vi "Read Step State.vi"(8 "error in (no error)":errorcluster, 11 "Base Step in":refnum<class "Base Step.lvclass">) -> (0 "error out":errorcluster, 2 "Step State":T1={"Result"="N/A", "Status"="IDLE", "Enabled"=TRUE, "Upper"="", "Target"="", "Lower"="", "Value"=""}, 3 "Base Step out":refnum<class "Base Step.lvclass">)   [LabVIEW 2024, in "Ramses Sequencer.lvlib" / "Base Step.lvclass"]
uses:
  Base Step.lvclass
  Typedefs/Step State.ctl
  Base Step.lvclass/Base Step.ctl
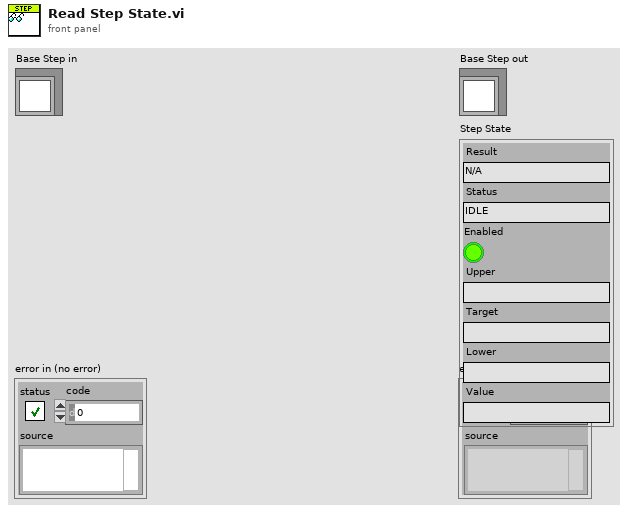
[diagram p1: front panel]
types:
  T1 = typedef "Ramses Sequencer.lvlib/Base Step.lvclass/Step State.ctl" = cluster{"Result":string, "Status":string, "Enabled":bool, "Upper":string, "Target":string, "Lower":string, "Value":string}
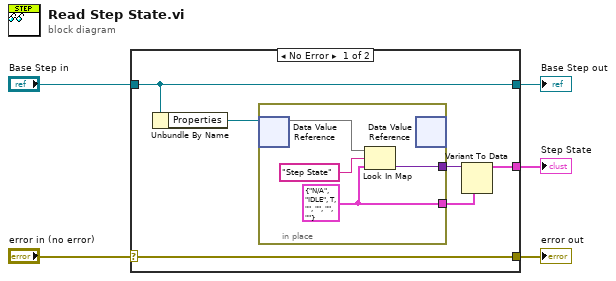
[diagram p0: block diagram]
diagram:
  n1 = case shown="No Error" "error in (no error)" {
    selector: "error in (no error)" -> [w11 w16]
    tunnel: [w11 w16] -> w4
    tunnel: [w10 w17] -> w2
    tunnel: "Base Step in" -> [w10 w17]
    tunnel: [w6 _] -> w1
    frame No Error {
      n2 = Unbundle By Name(w10) -> ("Properties"=w9:refnum<data-value>)
      n3 = in-place {
        in-place-border: [w13] -> w8
        in-place-border: [w12] -> w7
        w12 = T1 {"Result"="N/A", "Status"="IDLE", "Enabled"=TRUE, "Upper"="", "Target"="", "Lower"="", "Value"=""} ("Step State")
        n4 = in-place-dvr #1(w9) -> (w14:map{string, variant})  [unwired: 1 out]
        n5 = Look In Map(map=w14, key="Step State" ("Key"), default value=w12) -> (value=w13:variant)  [unwired: 1 out]
        n6 = in-place-dvr #1() -> ()  [unwired: 1 in, 2 out]
      }
      n7 = Variant To Data(type=w7, Variant=w8) -> (data=w6:T1)  [unwired: 1 in, 1 out]
    }
    frame Error {
    }
  }
  "error out" <- w4
  "Base Step out" <- w2
  "Step State" <- w1
